vi "AK Befehl Auswerten_v1.1.vi"(10 "Array":string[](array[string])) -> (2 "String für schreiben":string)   [LabVIEW 2020, in "AK-Schnittstelle.lvlib"]
uses:
  AK-Schnittstelle.lvlib
  Aktionen Stoernummern pruefen.ctl
  Aktionen Zustandsfehlerinformation.ctl
  Funktionstasten/Zustaende.ctl
  Funktionstasten/Funktionstasten.lvlib
  Funktionstasten/Betriebsart.ctl
  Funktionstasten/Funktionstasten-Aktion.ctl
  Aktionen Gespeicherte Werte.ctl
  Seiten/Log Konfig/LogKonfig.lvlib
  Seiten/Log Konfig/Aktionen Trigger.ctl
  Seiten/FT-IR/FT-IR.lvlib
  Seiten/FT-IR/FGV FT-IR Gasliste Aktionen.ctl
  Messdaten/Messdaten.lvlib
  Messdaten/Aktionen FGV Messdaten.ctl
  Seiten/System Einstellungen V2/System Einstellungen V2.lvlib
  Seiten/System Einstellungen V2/Aktioen FGV System Konstanten.ctl
  Seiten/Erweiterte Konfig/FGV PID Aktionen.ctl
  Seiten/Erweiterte Konfig/Erweiterte Konfig.lvlib
  Seiten/Erweiterte Konfig/Dichtheitstest.vi
  Allgemein/allgemeine Sub-VIs.lvlib
  cRIO/PC/Kommunikation mit cRIO.lvlib
  Seiten/FT-IR/FGV FT-IR Diagnose Aktionen.ctl
  Seiten/Erweiterte Konfig/Status Dichtheitstest Aktionen.ctl
  Seiten/System Einstellungen V2/Aktioen FGV System.ctl
  AK Namen Aktionen.ctl
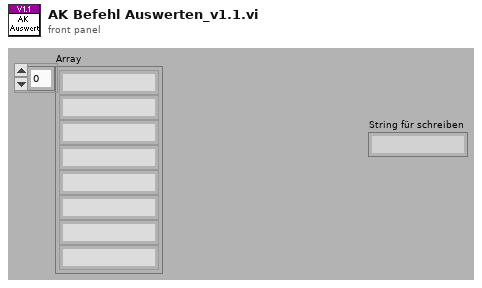
[diagram p1: front panel]
types:
  T1 = typedef "AK-Schnittstelle.lvlib/Aktionen Stoernummern pruefen.ctl" = enum16{"lesen", "prüfen"}
  T2 = typedef "AK-Schnittstelle.lvlib/Aktionen Zustandsfehlerinformation.ctl" = enum16{"OK", "Offline", "Busy", "Syntax Error", "Datenfehler"}
  T3 = typedef "AK-Schnittstelle.lvlib/AK Namen Aktionen.ctl" = enum16{"lesen", "laden", "speichern Namen", "AK Namen", "Liste erstellen", "EKFG erstellen", "speichern EKFG", "EKFG schreiben", "Neuen Eintrag erzeugen"}
  T4 = typedef "AK-Schnittstelle.lvlib/Aktionen Gespeicherte Werte.ctl" = enum16{"lesen", "laden", "speichern", "Seriell", "TCP", "Diverse", "AKTIV", "AK-Namen"}
  T5 = typedef "System Einstellungen V2.lvlib/Aktioen FGV System Konstanten.ctl" = enum16{"lesen", "laden", "speichern", "Sprache"}
  T6 = typedef "System Einstellungen V2.lvlib/Aktioen FGV System.ctl" = enum16{"lesen", "laden", "speichern", "Optionen schreiben", "Zeitstempel", "Reset BMP", "Reset SQP", "Wartung", "Werkseinstellung"}
  T7 = typedef "Messdaten.lvlib/Aktionen FGV Messdaten.ctl" = enum16{"lesen", "schreiben", "löschen", "Mittelwerte", "Komponente"}
  T8 = typedef "Funktionstasten.lvlib/Funktionstasten-Aktion.ctl" = enum16{"Initialisieren", "Zustand setzen", "Taste gedrückt", "Fehler speichern", "Lesen", "Manuell", "Remote", "Bitparallel", "Samplepoint", "Zeit Prüfen", "reset Umschalten"}
  T9 = typedef "FT-IR.lvlib/FGV FT-IR Gasliste Aktionen.ctl" = enum16{"lesen", "Gasliste FT-IR", "Gasliste ausgelesen", "laden", "speichern", "löschen"}
  T10 = typedef "FT-IR.lvlib/FGV FT-IR Diagnose Aktionen.ctl" = enum16{"Lesen", "Diagnose Schreiben", "Min Schreiben", "Max Schreiben"}
  T11 = typedef "Erweiterte Konfig.lvlib/Status Dichtheitstest Aktionen.ctl" = enum16{"lesen", "Zeitstempel", "Daten", "läuft", "Protokolldaten"}
  T12 = typedef "Funktionstasten.lvlib/Zustaende.ctl" = enum16{"Standby", "Pause", "Eco", "Messen", "Kalibrieren", "Spülen Filter", "Spülen Leitung", "Umgebungsluft", "0-Gas", "Cal-Gas", "CG zu PNS", "-------------", "Init 1", "Init 2", "Init 3", "Init 4", "Messen vorbereiten", "Messen durchführen", "Exit"}
  T13 = typedef "Funktionstasten.lvlib/Betriebsart.ctl" = enum16{"Manuell", "Remote", "Bitparallel"}
  T14 = typedef "Funktionstasten.lvlib/Zustaende.ctl" = enum16{"Standby", "Pause", "Eco", "Messen", "Kalibrieren", "Spülen Filter", "Spülen Leitung", "Umgebungsluft", "0-Gas", "Cal-Gas 1", "-------------", "Init 1", "Init 2", "Init 3", "Init 4", "Messen vorbereiten", "Messen durchführen", "Exit"}
  T15 = typedef "LogKonfig.lvlib/Aktionen Trigger.ctl" = enum16{"lesen", "ALLE schreiben", "Trigger prüfen", "Trigger rücksetzen"}
  T16 = typedef "Erweiterte Konfig.lvlib/FGV PID Aktionen.ctl" = enum16{"Lesen", "Schreiben PID", "Schreiben Sonstige", "Dichtheitstest", "Aktionen Dicht.", "Parameter Sensor"}
  T17 = typedef "AK-Schnittstelle.lvlib/Diverse gespeicherte Werte.ctl" = cluster{"Kalibriergaseingang":i16, "SamplePoint":i16, "CalGas zu PNS":i16, "Gas-Reihenfolge":i16[], "Zeit 0-Gas":sgl, "Zeit CalGas":sgl, "AK Befehlssatz":T18}
  T18 = typedef "AK-Schnittstelle.lvlib/AK Befehlssatz.ctl" = enum16{"MEXA", "IAG v1.4", "AVL (Puma)", "PEUS"}
  T19 = typedef "System Einstellungen.lvlib/Optionen.ctl" = cluster{"Störmeldep.":bool, "Betriebszustände":bool, "LN2 Befüllung":bool, "Klimaanlage ?":bool, "AK in ppm":bool, "log Cal-Gas":bool, "log 0-Gas":bool, "log CG zu PNS":bool, "Reserve":bool, "Reserve1":bool, "PNS?":bool, "Container":bool, "Mit N2 spülen":bool, "Span Gas Auswahl":T20}
  T20 = typedef "Funktionstasten.lvlib/Spaneingang.ctl" = u16
  T21 = typedef "String - Ausgabefeld.ctl" = string
  T22 = cluster{"AI0: Durchfluss FT-IR":sgl, "AI1: Druck Ausgang":sgl, "AI2: Umgebungsdruck":sgl, "AI3: Druck FT-IR":sgl, "AI4: Druck CalGas":sgl, "AI5: Reserve":sgl, "AI6: Reserve":sgl, "AI7: Reserve":sgl, "Rohwert Durchfluss FT-IR":sgl, "Rohwert Druck Ausgang":sgl, "Rohwert Umgebungsdruck":sgl, "Rohwert Druck FT-IR":sgl, "Rohwert Durchfluss M":sgl, "TC0: Schaltschrank":sgl, "TC1: Filter":sgl, "TC2: Pumpe":sgl, "TC3: HL BMP zu Filter":sgl, "TC4: HL zu FT-IR":sgl, "TC5: HL Extern SP1":sgl, "TC6: HL Extern SP2":sgl, "TC7: Heizung Extern 1":sgl, "TC8: Heizung Extern 2":sgl, "TC9: Reserve":sgl, "TC10: Reserve":sgl, "TC11: Reserve":sgl, "TC12: FT-IR":sgl, "TC13: Reserve":sgl, "TC14: Reserve":sgl, "TC15: Reserve":sgl}
  T23 = typedef "LogKonfig.lvlib/Element Triggerereignisse.ctl" = cluster{"Trigger verwenden":T24, "Messwert":u16, "kl./gr.":u16, "Wert":sgl, "Puffergröße":sgl}
  T24 = typedef "LogKonfig.lvlib/Auswahlfeld aktiviert-deaktiviert.ctl" = u16
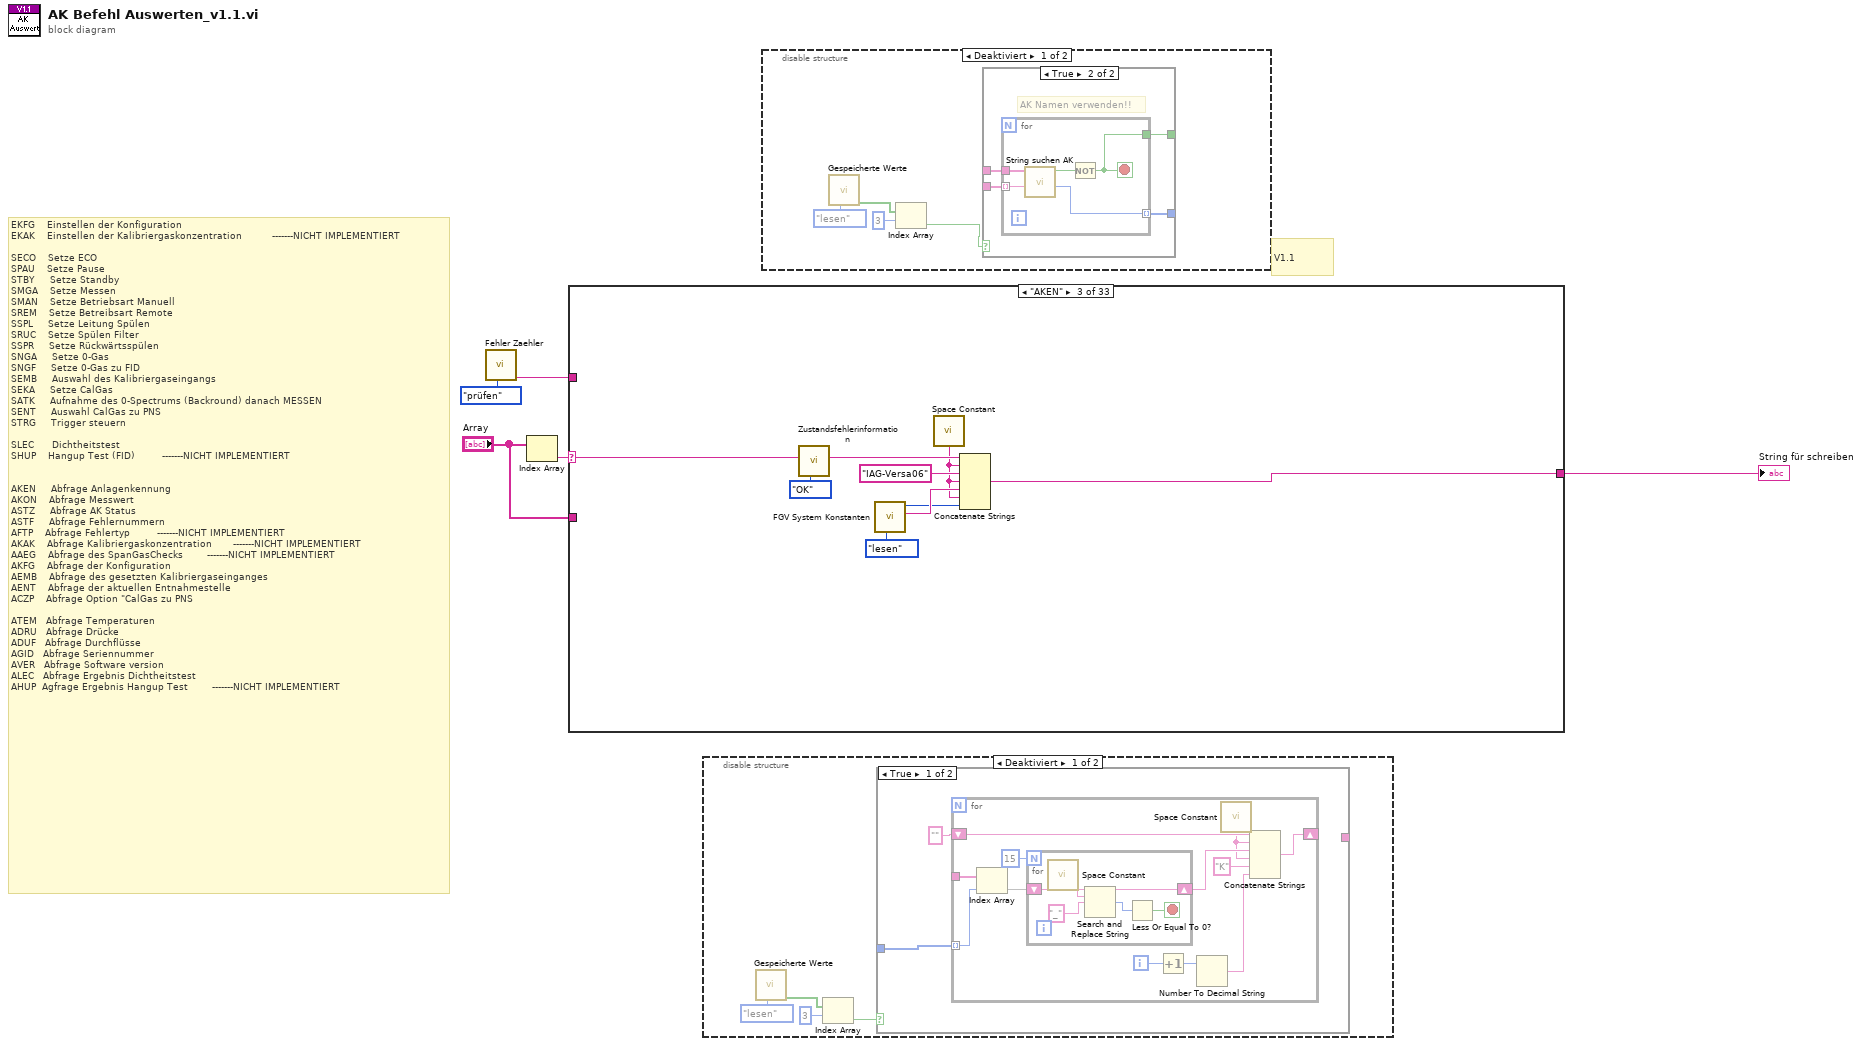
[diagram p0: block diagram]
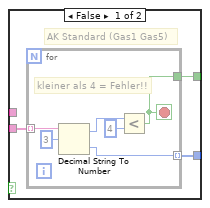
[diagram p2: hidden frame]
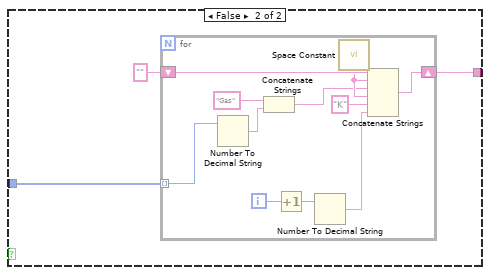
[diagram p4: hidden frame]
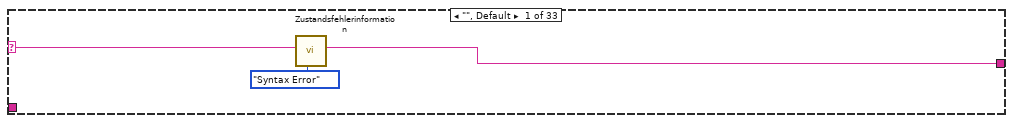
[diagram p6: hidden frame]
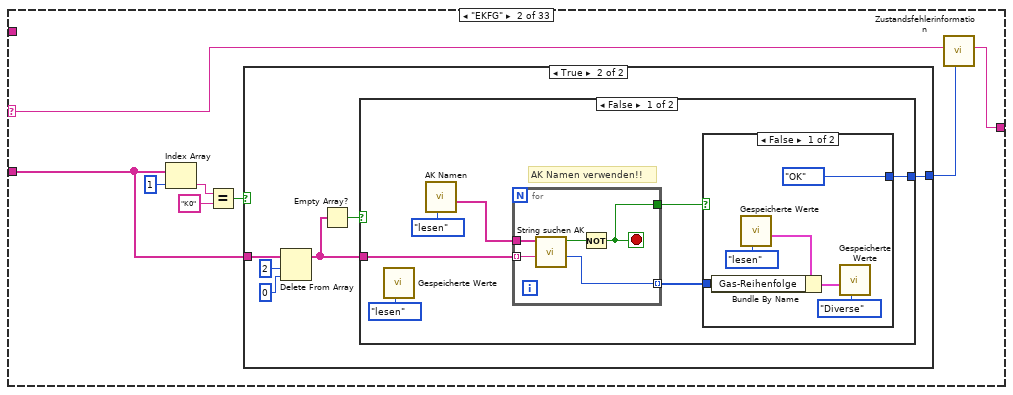
[diagram p7: hidden frame]
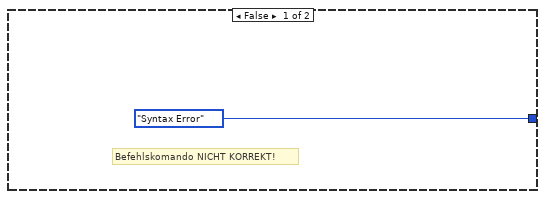
[diagram p8: hidden frame]
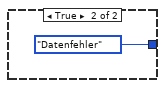
[diagram p9: hidden frame]
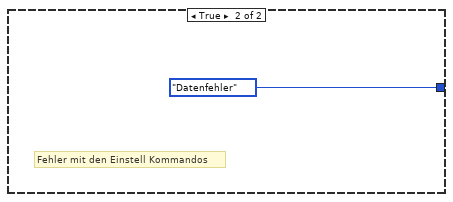
[diagram p10: hidden frame]
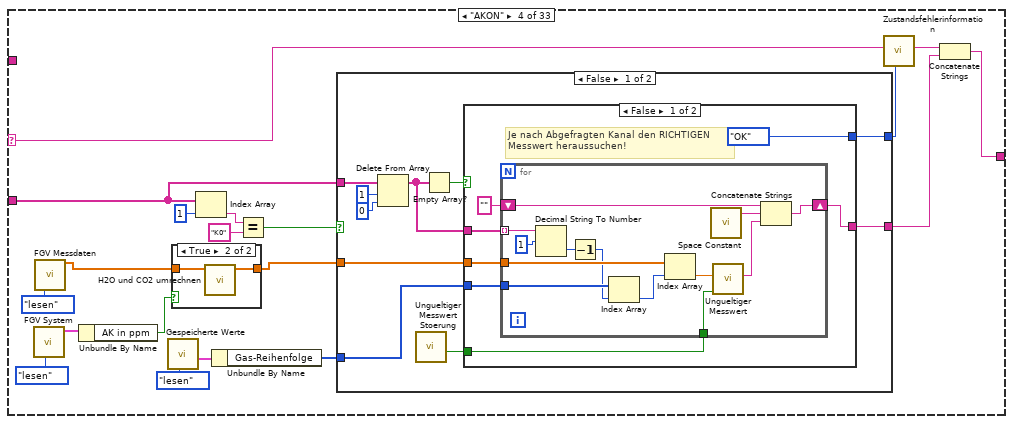
[diagram p11: hidden frame]
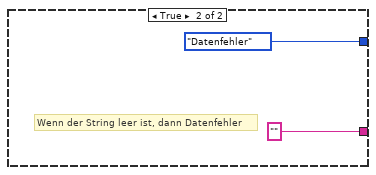
[diagram p13: hidden frame]
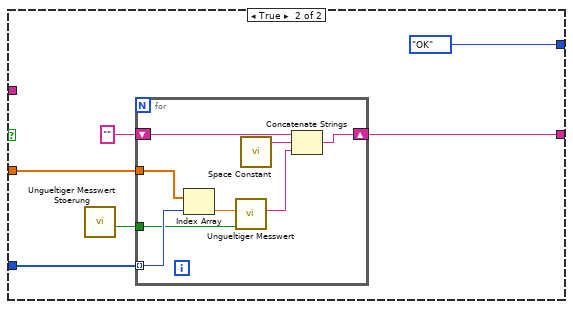
[diagram p14: hidden frame]
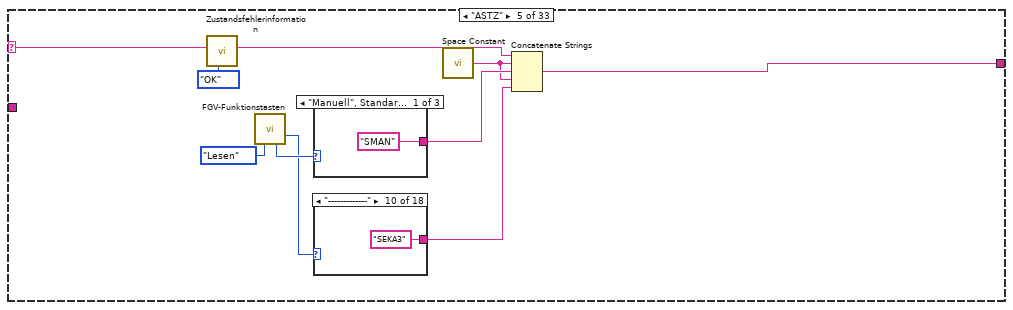
[diagram p15: hidden frame]
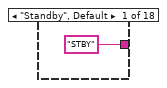
[diagram p16: hidden frame]
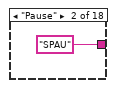
[diagram p17: hidden frame]
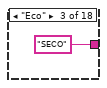
[diagram p18: hidden frame]
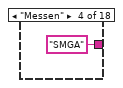
[diagram p19: hidden frame]
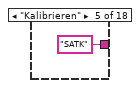
[diagram p20: hidden frame]
diagram:
  # "V1.1"
  # "EKFG    Einstellen der Konfiguration\nEKAK    Einstellen der Kalibriergaskonzentration          -------NICHT IMPLEMENTIERT\n\nSECO    Setze ECO\nSPAU    Setze Pause\nSTBY     Setze Standby\nSMGA    Setze Messen\nSMAN    Setze Betriebsart Manuell\nSREM    Setze Betreibsart Remote\nSSPL     Setze Leitung Spülen\nSRUC    Setze Spülen Filter\nSSPR     Setze Rückwärtsspülen\nSNGA     Setze 0-Gas\nSNGF     Setze 0-Gas zu FID\nSEMB     Auswahl des Kalibriergaseingangs\nSEKA     Setze CalGas\nSATK     Aufnahme des 0-Spectrums (Backround) danach MESSEN\nSENT     Auswahl CalGas zu PNS\nSTRG     Trigger steuern\n\nSLEC      Dichtheitstest\nSHUP    Hangup Test (FID)         -------NICHT IMPLEMENTIERT\n\n\nAKEN     Abfrage Anlagenkennung\nAKON    Abfrage Messwert\nASTZ     Abfrage AK Status\nASTF     Abfrage Fehlernummern\nAFTP    Abfrage Fehlertyp         -------NICHT IMPLEMENTIERT\nAKAK    Abfrage Kalibriergaskonzentration       -------NICHT IMPLEMENTIERT\nAAEG    Abfrage des SpanGasChecks        -------NICHT IMPLEMENTIERT\nAKFG    Abfrage der Konfiguration\nAEMB    Abfrage des gesetzten Kalibriergaseinganges\nAENT    Abfrage der aktuellen Entnahmestelle\nACZP    Abfrage Option \"CalGas zu PNS\n\nATEM   Abfrage Temperaturen\nADRU   Abfrage Drücke\nADUF   Abfrage Durchflüsse\nAGID   Abfrage Seriennummer\nAVER   Abfrage Software version\nALEC   Abfrage Ergebnis Dichtheitstest\nAHUP  Agfrage Ergebnis Hangup Test        -------NICHT IMPLEMENTIERT"
  n1 = call "Fehler Zaehler.vi"("Aktionen"=Aktionen_Stoernummern_pruefen."prüfen") -> ("Fehlerzähler"=w3:string)  [unwired: 7 in, 3 out]
  n2 = Index Array(array="Array") -> (element=w2:string)  [unwired: 1 in]
  n3 = case shown="\"AKEN\"" w2 {
    selector: w2 -> [w7 w15 w49 w70 w128 w148 w159 w189 w198 w207 w223 w246 w260 w267 w274 w289 w298 w301 w304 w307 w317 w327 w331 w341 w345 w347 w360 w365 w386 w405 w409 w431 w470]
    tunnel: [w6 w14 w51 w71 w130 w150 w161 w191 w200 w209 w211 w241 w257 w262 w270 w282 w297 w300 w303 w306 w316 w326 w330 w340 w344 w346 w359 w364 w385 w404 w408 w430 w469] -> w5
    tunnel: w3 -> [_ _ _ _ _ _ _ _ _ _ _ _ _ _ _ _ _ _ _ _ _ _ _ _ _ _ _ _ _ _ _ _ _]
    tunnel: "Array" -> [_ w16 _ w61 _ _ _ _ _ _ _ _ _ _ _ _ _ _ _ _ w309 w319 _ w339 _ _ _ w363 _ _ w407 w429 _]
    frame "", Default {
      n4 = call "Zustandsfehlerinformation.vi"("Aktionen"=Aktionen_Zustandsfehlerinformation."Syntax Error", "String"=w7) -> ("String"=w6:string)  [unwired: 9 in]
    }
    frame "EKFG" {
      n5 = Index Array(array=w16, index=1 ("Index")) -> (element=w12:string)
      n6 = Equal?(x=w12, y="K0") -> (x = y?=w10:bool)
      n7 = case shown="True" w10 {
        tunnel: w16 -> [_ w21]
        tunnel: [Aktionen_Zustandsfehlerinformation."Syntax Error" ("Aktionen") w18] -> w9
        frame False {
          # "Befehlskomando NICHT KORREKT!"
        }
        frame True {
          n8 = Delete From Array(array=w21, length=2 ("Länge"), index=0 ("Index")) -> (array with subset deleted=w20:string[])  [unwired: 1 out]
          n9 = Empty Array?(array=w20) -> (empty?=w19:bool)
          n10 = case shown="False" w19 {
            tunnel: w20 -> [w30 _]
            tunnel: [w27 Aktionen_Zustandsfehlerinformation."Datenfehler" ("Aktionen")] -> w18
            frame False {
              # "AK Namen verwenden!!"
              n11 = call "Gespeicherte Werte.vi"("Aktionen"=Aktionen_Gespeicherte_Werte."lesen") -> ()  [unwired: 6 in, 5 out]
              n12 = call "AK Namen.vi"("Aktionen"=AK_Namen_Aktionen."lesen") -> ("AK Namen"=w24:string[])  [unwired: 7 in, 3 out]
              n13 = for {
                tunnel: w30 -> [w33] mode=indexing
                tunnel: [w32] -> w29 mode=indexing
                tunnel: w24 -> [w34]
                tunnel: [w35] -> w26
                stop <- w35 stop-if-true
                n14 = call "String suchen AK.vi"("gesucht"=w33, "Namen"=w34) -> ("Index"=w32:i32, "Gefunden?"=w31:bool)  [unwired: 8 in]
                n15 = Not(x=w31) -> (.not. x?=w35:bool)
              }
              n16 = case shown="False" w26 {
                tunnel: w29 -> [w40 _]
                tunnel: [Aktionen_Zustandsfehlerinformation."OK" ("Aktionen") Aktionen_Zustandsfehlerinformation."Datenfehler" ("Aktionen")] -> w27
                frame False {
                  n17 = call "Gespeicherte Werte.vi"("Aktionen"=Aktionen_Gespeicherte_Werte."lesen") -> ("Diverse Werte"=w38:T17)  [unwired: 6 in, 4 out]
                  n18 = Bundle By Name(cluster=w38, "Gas-Reihenfolge"=w40) -> (w37:T17)
                  n19 = call "Gespeicherte Werte.vi"("Aktionen"=Aktionen_Gespeicherte_Werte."Diverse", "Diverse Werte"=w37) -> ()  [unwired: 5 in, 5 out]
                }
                frame True {
                }
              }
            }
            frame True {
              # "Fehler mit den Einstell Kommandos"
            }
          }
        }
      }
      n20 = call "Zustandsfehlerinformation.vi"("Aktionen"=w9, "String"=w15) -> ("String"=w14:string)  [unwired: 9 in]
    }
    frame "AKEN" {
      n21 = call "Zustandsfehlerinformation.vi"("Aktionen"=Aktionen_Zustandsfehlerinformation."OK", "String"=w49) -> ("String"=w48:string)  [unwired: 9 in]
      n22 = call "FGV System Konstanten.vi"("Aktionen"=Aktioen_FGV_System_Konstanten."lesen") -> ("LanguageList"=w46:string, "Sprachindex"=w44:u16)  [unwired: 6 in, 3 out]
      n23 = call <vilib>:"Space Constant.vi"() -> ("String"=w45:string)
      n24 = Concatenate Strings(w48, w45, "IAG-Versa06" ("String"), w45, w46, w45, w44) -> (w51:string)
    }
    frame "AKON" {
      n25 = call "FGV System.vi"("Aktionen"=Aktioen_FGV_System."lesen") -> ("Optionen"=w55:T19)  [unwired: 8 in, 2 out]
      n26 = call "FGV Messdaten.vi"("Aktionen"=Aktionen_FGV_Messdaten."lesen") -> ("Aktuelle Messwerte"=w57:sgl[])  [unwired: 6 in, 8 out]
      n27 = Unbundle By Name(w55) -> ("AK in ppm"=w53:bool)
      n28 = call "Gespeicherte Werte.vi"("Aktionen"=Aktionen_Gespeicherte_Werte."lesen") -> ("Diverse Werte"=w59:T17)  [unwired: 6 in, 4 out]
      n29 = case shown="True" w53 {
        tunnel: w57 -> [w72 w74]
        tunnel: [w72 w73] -> w56
        frame False {
        }
        frame True {
          n30 = call "H2O und CO2 umrechnen.vi"("Aktuelle Messwerte"=w74) -> ("Aktuelle Messwerte"=w73:sgl[])  [unwired: 10 in]
        }
      }
      n31 = Index Array(array=w61, index=1 ("Index")) -> (element=w64:string)
      n32 = Unbundle By Name(w59) -> ("Gas-Reihenfolge"=w67:i16[])
      n33 = Equal?(x=w64, y="K0") -> (x = y?=w62:bool)
      n34 = case shown="False" w62 {
        tunnel: w67 -> [w78 w112]
        tunnel: [w76 w110] -> w66
        tunnel: w56 -> [w77 w109]
        tunnel: w61 -> [w82 _]
        tunnel: [w80 Aktionen_Zustandsfehlerinformation."OK" ("Aktionen")] -> w60
        frame False {
          n35 = Delete From Array(array=w82, length=1 ("Länge"), index=0 ("Index")) -> (array with subset deleted=w79:string[])  [unwired: 1 out]
          n36 = call "Ungueltiger Messwert Stoerung.vi"() -> ("Störung Messgerät"=w75:bool)  [unwired: 11 in]
          n37 = Empty Array?(array=w79) -> (empty?=w81:bool)
          n38 = case shown="False" w81 {
            tunnel: [Aktionen_Zustandsfehlerinformation."OK" ("Aktionen") Aktionen_Zustandsfehlerinformation."Datenfehler" ("Aktionen")] -> w80
            tunnel: w79 -> [w90 _]
            tunnel: w78 -> [w89 _]
            tunnel: w77 -> [w88 _]
            tunnel: [w87 ""] -> w76
            tunnel: w75 -> [w85 _]
            frame False {
              # "Je nach Abgefragten Kanal den RICHTIGEN\nMesswert heraussuchen!"
              n39 = for {
                tunnel: w90 -> [w104] mode=indexing
                tunnel: w89 -> [w102]
                tunnel: w88 -> [w101]
                shift-right: [w100] -> w87
                shift-left: "" -> [w99]
                tunnel: w85 -> [w93]
                n40 = Decimal String To Number(string=w104, offset=1 ("Offset (0)")) -> (number=w98:i32)  [unwired: 1 in, 1 out]
                n41 = Decrement(x=w98) -> (x-1=w97:i32)
                n42 = Index Array(array=w102, index=w97) -> (element=w95:i16)
                n43 = Index Array(array=w101, index=w95) -> (element=w94:sgl)
                n44 = call <vilib>:"Space Constant.vi"() -> ("String"=w96:string)
                n45 = call "Ungueltiger Messwert.vi"("Stöung Messgerät"=w93, "Messwert"=w94) -> ("Messwert String"=w92:string)  [unwired: 9 in]
                n46 = Concatenate Strings(w99, w96, w92) -> (w100:string)
              }
            }
            frame True {
              # "Wenn der String leer ist, dann Datenfehler"
            }
          }
        }
        frame True {
          n47 = call "Ungueltiger Messwert Stoerung.vi"() -> ("Störung Messgerät"=w107:bool)  [unwired: 11 in]
          n48 = for {
            tunnel: w112 -> [w116] mode=indexing
            shift-right: [w120] -> w110
            shift-left: "" -> [w119]
            tunnel: w109 -> [w118]
            tunnel: w107 -> [w114]
            n49 = Index Array(array=w118, index=w116) -> (element=w115:sgl)
            n50 = call "Ungueltiger Messwert.vi"("Stöung Messgerät"=w114, "Messwert"=w115) -> ("Messwert String"=w113:string)  [unwired: 9 in]
            n51 = call <vilib>:"Space Constant.vi"() -> ("String"=w117:string)
            n52 = Concatenate Strings(w119, w117, w113) -> (w120:string)
          }
        }
      }
      n53 = call "Zustandsfehlerinformation.vi"("Aktionen"=w60, "String"=w70) -> ("String"=w69:string)  [unwired: 9 in]
      n54 = Concatenate Strings(w69, w66) -> (w71:string)
    }
    frame "ASTZ" {
      n55 = call "Zustandsfehlerinformation.vi"("Aktionen"=Aktionen_Zustandsfehlerinformation."OK", "String"=w128) -> ("String"=w127:string)  [unwired: 9 in]
      n56 = call "FGV-Funktionstasten.vi"("Aktion"=Funktionstasten-Aktion."Lesen") -> ("ausgewählte Funktion"=w123:T12, "Betriebsart"=w125:T13)  [unwired: 7 in, 6 out]
      n57 = case shown="\"Manuell\", Standard" w125 {
        tunnel: ["SMAN" ("String") "SREM" ("String") "SBIT" ("String")] -> w124
        frame "Manuell", Default {
        }
        frame "Remote" {
        }
        frame "Bitparallel" {
        }
      }
      n58 = case shown="\"-------------\"" w123 {
        tunnel: ["STBY" ("String") "SPAU" ("String") "SECO" ("String") "SMGA" ("String") "SATK" ("String") "SRUC" ("String") "SSPL" ("String") "SNGA" ("String") "SEKA1" ("String") "SEKA3" ("String") _ _ _ _ _ _ _ _] -> w121
        frame "Standby", Default {
        }
        frame "Pause" {
        }
        frame "Eco" {
        }
        frame "Messen" {
        }
        frame "Kalibrieren" {
        }
        frame "Spülen Filter" {
        }
        frame "Spülen Leitung" {
        }
        frame "0-Gas" {
        }
        frame "Cal-Gas" {
        }
        frame "-------------" {
        }
        frame "-------------" {
        }
        frame "Init 1" {
        }
        frame "Init 2" {
        }
        frame "Init 3" {
        }
        frame "Init 4" {
        }
        frame "Messen vorbereiten" {
        }
        frame "Messen durchführen" {
        }
        frame "Exit" {
        }
      }
      n59 = call <vilib>:"Space Constant.vi"() -> ("String"=w122:string)
      n60 = Concatenate Strings(w127, w122, w124, w122, w121) -> (w130:string)
    }
    frame "ASTF" {
      n61 = call "Zustandsfehlerinformation.vi"("Aktionen"=Aktionen_Zustandsfehlerinformation."OK", "String"=w148) -> ("String"=w147:string)  [unwired: 9 in]
      n62 = call "Fehler Zaehler.vi"("Aktionen"=Aktionen_Stoernummern_pruefen."lesen") -> ("Fehler Nummern"=w145:string)  [unwired: 7 in, 3 out]
      n63 = call <vilib>:"Space Constant.vi"() -> ("String"=w144:string)
      n64 = Concatenate Strings(w147, w144, w145) -> (w150:string)
    }
    frame "AKFG" {
      n65 = call "Gespeicherte Werte.vi"("Aktionen"=Aktionen_Gespeicherte_Werte."lesen") -> ("Diverse Werte"=w156:T17)  [unwired: 6 in, 4 out]
      n66 = Unbundle By Name(w156) -> ("Gas-Reihenfolge"=w154:i16[])
      n67 = disable-structure shown="Deaktiviert" {
        disable-tunnel: [w180 _] -> _
        frame Disabled {
          n68 = call "FGV Gasliste.vi"("Aktionen"=FGV_FT-IR_Gasliste_Aktionen."lesen") -> ("Aktuelle Gasliste gesamt"=w180:T21[])  [unwired: 8 in, 2 out]
        }
        frame Enabled {
        }
      }
      n69 = call "AK Namen.vi"("Aktionen"=AK_Namen_Aktionen."lesen") -> ("AK Namen"=w151:string[])  [unwired: 7 in, 3 out]
      n70 = for {
        tunnel: w154 -> [w170] mode=indexing
        shift-right: [w173] -> w153
        shift-left: "" -> [w172]
        tunnel: w151 -> [w171]
        i -> [w163]
        n71 = Index Array(array=w171, index=w170) -> (element=w168:string)
        n72 = for {
          N: 15 -> [_]
          shift-right: [w178] -> w167
          shift-left: w168 -> [w179]
          stop <- w176 stop-if-true
          n73 = call <vilib>:"Space Constant.vi"() -> ("String"=w175:string)
          n74 = Search and Replace String(input string=w179, search string=w175, replace string="_") -> (result string=w178:string, number of replacements=w177:i32)  [unwired: 5 in, 2 out]
          n75 = Less Or Equal To 0?(x=w177) -> (x <= 0?=w176:bool)
        }
        n76 = Increment(x=w163) -> (x+1=w165:i32)
        n77 = Number To Decimal String(number=w165) -> (decimal integer string=w162:string)  [unwired: 1 in]
        n78 = call <vilib>:"Space Constant.vi"() -> ("String"=w166:string)
        n79 = Concatenate Strings(w172, w166, w167, w166, "K" ("String"), w162) -> (w173:string)
      }
      n80 = call "Zustandsfehlerinformation.vi"("Aktionen"=Aktionen_Zustandsfehlerinformation."OK", "String"=w159) -> ("String"=w158:string)  [unwired: 9 in]
      n81 = Concatenate Strings(w158, w153) -> (w161:string)
    }
    frame "AEMB" {
      n82 = call "Zustandsfehlerinformation.vi"("Aktionen"=Aktionen_Zustandsfehlerinformation."OK", "String"=w189) -> ("String"=w188:string)  [unwired: 9 in]
      n83 = call "Gespeicherte Werte.vi"("Aktionen"=Aktionen_Gespeicherte_Werte."lesen") -> ("Diverse Werte"=w182:T17)  [unwired: 6 in, 4 out]
      n84 = Unbundle By Name(w182) -> ("Kalibriergaseingang"=w186:i16)
      n85 = call <vilib>:"Space Constant.vi"() -> ("String"=w183:string)
      n86 = Number To Decimal String(number=w186) -> (decimal integer string=w184:string)  [unwired: 1 in]
      n87 = Concatenate Strings(w188, w183, "M" ("String"), w184) -> (w191:string)
    }
    frame "AENT" {
      n88 = call "Zustandsfehlerinformation.vi"("Aktionen"=Aktionen_Zustandsfehlerinformation."OK", "String"=w198) -> ("String"=w197:string)  [unwired: 9 in]
      n89 = call "FGV-Funktionstasten.vi"("Aktion"=Funktionstasten-Aktion."Lesen") -> ("Samplepoint"=w192:u16)  [unwired: 7 in, 7 out]
      n90 = call <vilib>:"Space Constant.vi"() -> ("String"=w194:string)
      n91 = Number To Decimal String(number=w192) -> (decimal integer string=w195:string)  [unwired: 1 in]
      n92 = Concatenate Strings(w197, w194, "M" ("String"), w195) -> (w200:string)
    }
    frame "ACZP" {
      n93 = call "Zustandsfehlerinformation.vi"("Aktionen"=Aktionen_Zustandsfehlerinformation."OK", "String"=w207) -> ("String"=w206:string)  [unwired: 9 in]
      n94 = call "Gespeicherte Werte.vi"("Aktionen"=Aktionen_Gespeicherte_Werte."lesen") -> ("Diverse Werte"=w201:T17)  [unwired: 6 in, 4 out]
      n95 = Unbundle By Name(w201) -> ("CalGas zu PNS"=w204:i16)
      n96 = call <vilib>:"Space Constant.vi"() -> ("String"=w202:string)
      n97 = Number To Decimal String(number=w204) -> (decimal integer string=w203:string)  [unwired: 1 in]
      n98 = Concatenate Strings(w206, w202, w203) -> (w209:string)
    }
    frame "ATEM" {
      n99 = call "Zustandsfehlerinformation.vi"("Aktionen"=Aktionen_Zustandsfehlerinformation."OK", "String"=w223) -> ("String"=w210:string)  [unwired: 9 in]
      n100 = call "FGV cRIO-Daten.vi"("Aktion"=enum16{"lesen", "schreiben"}."lesen") -> ("Analog Input"=w221:T22)  [unwired: 6 in, 8 out]
      n101 = Unbundle By Name(w221) -> ("TC1: Filter"=w218:sgl, "TC2: Pumpe"=w217:sgl, "TC3: HL BMP zu Filter"=w216:sgl, "TC4: HL zu FT-IR"=w215:sgl, "TC5: HL Extern SP1"=w214:sgl, "TC0: Schaltschrank"=w213:sgl)
      n102 = call "FGV FT-IR Diagnosewerte.vi"("Aktionen"=FGV_FT-IR_Diagnose_Aktionen."Lesen") -> ("Temperatur"=w219:dbl)  [unwired: 5 in, 5 out]
      n103 = Build Array(w219, w218, w217, w216, w215, w214, w213) -> (w212:dbl[])
      n104 = for {
        tunnel: w212 -> [w230] mode=indexing
        shift-right: [w225] -> w211
        shift-left: w210 -> [w228]
        n105 = Number To Fractional String(number=w230, precision (6)=i16 1 ("Genauigkeit (6)")) -> (F-format string=w226:string)  [unwired: 2 in]
        n106 = call <vilib>:"Space Constant.vi"() -> ("String"=w227:string)
        n107 = Concatenate Strings(w228, w227, w226) -> (w225:string)
      }
    }
    frame "ADRU" {
      n108 = call "Zustandsfehlerinformation.vi"("Aktionen"=Aktionen_Zustandsfehlerinformation."OK", "String"=w246) -> ("String"=w240:string)  [unwired: 9 in]
      n109 = call "FGV cRIO-Daten.vi"("Aktion"=enum16{"lesen", "schreiben"}."lesen") -> ("Analog Input"=w244:T22)  [unwired: 6 in, 8 out]
      n110 = Unbundle By Name(w244) -> ("AI1: Druck Ausgang"=w236:sgl, "AI4: Druck CalGas"=w234:sgl)
      n111 = call "FGV FT-IR Diagnosewerte.vi"("Aktionen"=FGV_FT-IR_Diagnose_Aktionen."Lesen") -> ("Druck"=w238:dbl)  [unwired: 5 in, 5 out]
      n112 = Number To Fractional String(number=w238, precision (6)=i16 3 ("Genauigkeit (6)")) -> (F-format string=w233:string)  [unwired: 2 in]
      n113 = Number To Fractional String(number=w236, precision (6)=i16 0 ("Genauigkeit (6)")) -> (F-format string=w231:string)  [unwired: 2 in]
      n114 = Number To Fractional String(number=w234, precision (6)=i16 1 ("Genauigkeit (6)")) -> (F-format string=w232:string)  [unwired: 2 in]
      n115 = Build Array(w233, w231, w232) -> (w242:string[])
      n116 = for {
        tunnel: w242 -> [w248] mode=indexing
        shift-right: [w249] -> w241
        shift-left: w240 -> [w251]
        n117 = call <vilib>:"Space Constant.vi"() -> ("String"=w250:string)
        n118 = Concatenate Strings(w251, w250, w248) -> (w249:string)
      }
    }
    frame "ADUF" {
      n119 = call "Zustandsfehlerinformation.vi"("Aktionen"=Aktionen_Zustandsfehlerinformation."OK", "String"=w260) -> ("String"=w256:string)  [unwired: 9 in]
      n120 = call "FGV cRIO-Daten.vi"("Aktion"=enum16{"lesen", "schreiben"}."lesen") -> ("Analog Input"=w259:T22)  [unwired: 6 in, 8 out]
      n121 = Unbundle By Name(w259) -> ("AI0: Durchfluss FT-IR"=w255:sgl)
      n122 = Number To Fractional String(number=w255, precision (6)=i16 1 ("Genauigkeit (6)")) -> (F-format string=w252:string)  [unwired: 2 in]
      n123 = call <vilib>:"Space Constant.vi"() -> ("String"=w253:string)
      n124 = Concatenate Strings(w256, w253, w252) -> (w257:string)
    }
    frame "AGID" {
      n125 = call "Zustandsfehlerinformation.vi"("Aktionen"=Aktionen_Zustandsfehlerinformation."OK", "String"=w267) -> ("String"=w264:string)  [unwired: 9 in]
      n126 = call "FGV System Konstanten.vi"("Aktionen"=Aktioen_FGV_System_Konstanten."lesen") -> ("LanguageList"=w263:string)  [unwired: 6 in, 4 out]
      n127 = call <vilib>:"Space Constant.vi"() -> ("String"=w266:string)
      n128 = Concatenate Strings(w264, w266, w263) -> (w262:string)
    }
    frame "AVER" {
      n129 = call "Zustandsfehlerinformation.vi"("Aktionen"=Aktionen_Zustandsfehlerinformation."OK", "String"=w274) -> ("String"=w271:string)  [unwired: 9 in]
      n130 = call "FGV System Konstanten.vi"("Aktionen"=Aktioen_FGV_System_Konstanten."lesen") -> ("Sprachindex"=w269:u16)  [unwired: 6 in, 4 out]
      n131 = call <vilib>:"Space Constant.vi"() -> ("String"=w273:string)
      n132 = Concatenate Strings(w271, w273, w269) -> (w270:string)
    }
    frame "ALEC" {
      n133 = call "Zustandsfehlerinformation.vi"("Aktionen"=Aktionen_Zustandsfehlerinformation."OK", "String"=w289) -> ("String"=w288:string)  [unwired: 9 in]
      n134 = call "Status Dichtheitstest.vi"("Aktionen"=Status_Dichtheitstest_Aktionen."lesen") -> ("Fehler"=w277:bool, "läuft?"=w281:bool, "Anstieg"=w286:sgl)  [unwired: 6 in, 2 out]
      n135 = Or(x=w281, y=w277) -> (x .or. y?=w280:bool)
      n136 = Number To Decimal String(number=w286) -> (decimal integer string=w285:string)  [unwired: 1 in]
      n137 = call <vilib>:"Space Constant.vi"() -> ("String"=w284:string)
      n138 = Concatenate Strings(w288, w284, w285) -> (w283:string)
      n139 = Select(t="error", s=w277, f="busy") -> (s? t:f=w276:string)
      n140 = case shown="True" w280 {
        tunnel: w283 -> [w291 w294]
        tunnel: [w291 w292] -> w282
        tunnel: w276 -> [_ w293]
        frame False {
        }
        frame True {
          n141 = call <vilib>:"Space Constant.vi"() -> ("String"=w295:string)
          n142 = Concatenate Strings(w294, w295, w293) -> (w292:string)
        }
      }
    }
    frame "SECO" {
      n143 = call "Setze Zustand.vi"("AK Befehl"=w298, "Zustand"=Zustaende."Eco") -> ("Antwort String"=w297:string)  [unwired: 8 in, 1 out]
    }
    frame "SPAU" {
      n144 = call "Setze Zustand.vi"("AK Befehl"=w301, "Zustand"=Zustaende."Pause") -> ("Antwort String"=w300:string)  [unwired: 8 in, 1 out]
    }
    frame "STBY" {
      n145 = call "Setze Zustand.vi"("AK Befehl"=w304, "Zustand"=Zustaende."Standby") -> ("Antwort String"=w303:string)  [unwired: 8 in, 1 out]
    }
    frame "SMGA" {
      n146 = call "Setze Zustand.vi"("AK Befehl"=w307, "Zustand"=Zustaende."Messen") -> ("Antwort String"=w306:string)  [unwired: 8 in, 1 out]
    }
    frame "SSPL" {
      n147 = Index Array(array=w309, index=2 ("Index")) -> (element=w313:string)
      n148 = Decimal String To Number(string=w313) -> (number=w312:i32)  [unwired: 2 in, 1 out]
      n149 = Divide(x=w312, y=10) -> (x/y=w310:dbl)
      n150 = To Single Precision Float(number=w310) -> (single precision float=w308:sgl)
      n151 = call "Setze Zustand.vi"("Zeit"=w308, "AK Befehl"=w317, "Zustand"=Zustaende."Spülen Leitung") -> ("Antwort String"=w316:string)  [unwired: 7 in, 1 out]
    }
    frame "SRUC" {
      n152 = Index Array(array=w319, index=2 ("Index")) -> (element=w323:string)
      n153 = Decimal String To Number(string=w323) -> (number=w322:i32)  [unwired: 2 in, 1 out]
      n154 = Divide(x=w322, y=10) -> (x/y=w320:dbl)
      n155 = To Single Precision Float(number=w320) -> (single precision float=w318:sgl)
      n156 = call "Setze Zustand.vi"("Zeit"=w318, "AK Befehl"=w327, "Zustand"=Zustaende."Spülen Filter") -> ("Antwort String"=w326:string)  [unwired: 7 in, 1 out]
    }
    frame "SSPR" {
      n157 = call "Setze Zustand.vi"("Befehl nicht vorhanden!"=TRUE, "AK Befehl"=w331, "Zustand"=Zustaende."Standby") -> ("Antwort String"=w330:string)  [unwired: 7 in, 1 out]
    }
    frame "SNGA" {
      n158 = Index Array(array=w339, index=2 ("Index")) -> (element=w337:string)
      n159 = Decimal String To Number(string=w337) -> (number=w336:i32)  [unwired: 2 in, 1 out]
      n160 = Divide(x=w336, y=10) -> (x/y=w334:dbl)
      n161 = To Single Precision Float(number=w334) -> (single precision float=w332:sgl)
      n162 = call "Setze Zustand.vi"("Zeit"=w332, "AK Befehl"=w341, "Zustand"=Zustaende."0-Gas") -> ("Antwort String"=w340:string)  [unwired: 7 in, 1 out]
    }
    frame "SNGF" {
      n163 = call "Setze Zustand.vi"("Befehl nicht vorhanden!"=TRUE, "AK Befehl"=w345, "Zustand"=Zustaende."Standby") -> ("Antwort String"=w344:string)  [unwired: 7 in, 1 out]
    }
    frame "SMAN" {
      n164 = call "FGV-Funktionstasten.vi"("Aktion"=Funktionstasten-Aktion."Lesen") -> ("Betriebsart"=w351:T13)  [unwired: 7 in, 7 out]
      n165 = Equal?(x=w351, y=Betriebsart."Remote" ("Betriebsart")) -> (x = y?=w348:bool)
      n166 = case shown="True" w348 {
        tunnel: w347 -> [w354 w357]
        tunnel: [w352 w356] -> w346
        frame False {
          n167 = call "Zustandsfehlerinformation.vi"("Aktionen"=Aktionen_Zustandsfehlerinformation."Offline", "String"=w354) -> ("String"=w352:string)  [unwired: 9 in]
        }
        frame True {
          n168 = call "Zustandsfehlerinformation.vi"("Aktionen"=Aktionen_Zustandsfehlerinformation."OK", "String"=w357) -> ("String"=w356:string)  [unwired: 9 in]
          n169 = call "FGV-Funktionstasten.vi"("Aktion"=Funktionstasten-Aktion."Manuell") -> ()  [unwired: 7 in, 8 out]
        }
      }
    }
    frame "SREM" {
      n170 = call "Zustandsfehlerinformation.vi"("Aktionen"=Aktionen_Zustandsfehlerinformation."OK", "String"=w360) -> ("String"=w359:string)  [unwired: 9 in]
      n171 = call "FGV-Funktionstasten.vi"("Aktion"=Funktionstasten-Aktion."Remote") -> ()  [unwired: 7 in, 8 out]
    }
    frame "SEMB" {
      n172 = call "FGV-Funktionstasten.vi"("Aktion"=Funktionstasten-Aktion."Lesen") -> ("Betriebsart"=w368:T13)  [unwired: 7 in, 7 out]
      n173 = Equal?(x=w368, y=Betriebsart."Remote" ("Betriebsart")) -> (x = y?=w369:bool)
      n174 = case shown="True" w369 {
        tunnel: w365 -> [w371 w383]
        tunnel: [w370 w382] -> w364
        tunnel: w363 -> [_ w381]
        frame False {
          n175 = call "Zustandsfehlerinformation.vi"("Aktionen"=Aktionen_Zustandsfehlerinformation."Offline", "String"=w371) -> ("String"=w370:string)  [unwired: 9 in]
        }
        frame True {
          n176 = Index Array(array=w381, index=2 ("Index")) -> (element=w379:string)
          n177 = call "Zustandsfehlerinformation.vi"("Aktionen"=Aktionen_Zustandsfehlerinformation."OK", "String"=w383) -> ("String"=w382:string)  [unwired: 9 in]
          n178 = Decimal String To Number(string=w379, offset=1 ("Offset (0)")) -> (number=w375:i32)  [unwired: 1 in, 1 out]
          n179 = call "Gespeicherte Werte.vi"("Aktionen"=Aktionen_Gespeicherte_Werte."lesen") -> ("Diverse Werte"=w374:T17)  [unwired: 6 in, 4 out]
          n180 = Bundle By Name(cluster=w374, "Kalibriergaseingang"=w375) -> (w373:T17)
          n181 = call "Gespeicherte Werte.vi"("Aktionen"=Aktionen_Gespeicherte_Werte."Diverse", "Diverse Werte"=w373) -> ()  [unwired: 5 in, 5 out]
        }
      }
    }
    frame "SEKA" {
      n182 = call "FGV-Funktionstasten.vi"("Aktion"=Funktionstasten-Aktion."Lesen") -> ("Betriebsart"=w389:T13)  [unwired: 7 in, 7 out]
      n183 = Equal?(x=w389, y=Betriebsart."Remote" ("Betriebsart")) -> (x = y?=w390:bool)
      n184 = case shown="True" w390 {
        tunnel: w386 -> [w392 w396]
        tunnel: [w391 w395] -> w385
        frame False {
          n185 = call "Zustandsfehlerinformation.vi"("Aktionen"=Aktionen_Zustandsfehlerinformation."Offline", "String"=w392) -> ("String"=w391:string)  [unwired: 9 in]
        }
        frame True {
          n186 = call "Gespeicherte Werte.vi"("Aktionen"=Aktionen_Gespeicherte_Werte."lesen") -> ("Diverse Werte"=w398:T17)  [unwired: 6 in, 4 out]
          n187 = Unbundle By Name(w398) -> ("Kalibriergaseingang"=w397:i16)
          n188 = case shown="3" w397 {
            tunnel: [Zustaende."Standby" ("Zustand") Zustaende."Cal-Gas 1" ("Zustand") Zustaende."-------------" ("Zustand") Zustaende."Init 1" ("Zustand")] -> w394
            frame 0, Default {
            }
            frame 1 {
            }
            frame 2 {
            }
            frame 3 {
            }
          }
          n189 = call "Setze Zustand.vi"("AK Befehl"=w396, "Zustand"=w394) -> ("Antwort String"=w395:string)  [unwired: 8 in, 1 out]
        }
      }
    }
    frame "SATK" {
      n190 = call "Setze Zustand.vi"("AK Befehl"=w405, "Zustand"=Zustaende."Kalibrieren") -> ("Antwort String"=w404:string)  [unwired: 8 in, 1 out]
    }
    frame "SENT" {
      n191 = call "FGV-Funktionstasten.vi"("Aktion"=Funktionstasten-Aktion."Lesen") -> ("Betriebsart"=w412:T13)  [unwired: 7 in, 7 out]
      n192 = Equal?(x=w412, y=Betriebsart."Remote" ("Betriebsart")) -> (x = y?=w413:bool)
      n193 = case shown="True" w413 {
        tunnel: w409 -> [w415 w427]
        tunnel: [w414 w426] -> w408
        tunnel: w407 -> [_ w425]
        frame False {
          n194 = call "Zustandsfehlerinformation.vi"("Aktionen"=Aktionen_Zustandsfehlerinformation."Offline", "String"=w415) -> ("String"=w414:string)  [unwired: 9 in]
        }
        frame True {
          n195 = Index Array(array=w425, index=2 ("Index")) -> (element=w423:string)
          n196 = call "Zustandsfehlerinformation.vi"("Aktionen"=Aktionen_Zustandsfehlerinformation."OK", "String"=w427) -> ("String"=w426:string)  [unwired: 9 in]
          n197 = Decimal String To Number(string=w423) -> (number=w417:i32)  [unwired: 2 in, 1 out]
          n198 = call "FGV-Funktionstasten.vi"("Samplepoint"=w417, "Aktion"=Funktionstasten-Aktion."Samplepoint") -> ()  [unwired: 6 in, 8 out]
          n199 = call "Gespeicherte Werte.vi"("Aktionen"=Aktionen_Gespeicherte_Werte."lesen") -> ("Diverse Werte"=w420:T17)  [unwired: 6 in, 4 out]
          n200 = Bundle By Name(cluster=w420, "SamplePoint"=w417) -> (w419:T17)
          n201 = call "Gespeicherte Werte.vi"("Aktionen"=Aktionen_Gespeicherte_Werte."Diverse", "Diverse Werte"=w419) -> ()  [unwired: 5 in, 5 out]
        }
      }
    }
    frame "STRG" {
      n202 = call "FGV-Funktionstasten.vi"("Aktion"=Funktionstasten-Aktion."Lesen") -> ("Betriebsart"=w434:T13)  [unwired: 7 in, 7 out]
      n203 = Equal?(x=w434, y=Betriebsart."Remote" ("Betriebsart")) -> (x = y?=w435:bool)
      n204 = case shown="False" w435 {
        tunnel: w431 -> [w437 w444]
        tunnel: [w436 w443] -> w430
        tunnel: w429 -> [_ w442]
        frame False {
          n205 = call "Zustandsfehlerinformation.vi"("Aktionen"=Aktionen_Zustandsfehlerinformation."Offline", "String"=w437) -> ("String"=w436:string)  [unwired: 9 in]
        }
        frame True {
          n206 = Index Array(array=w442, index=2 ("Index")) -> (element=w440:string)
          n207 = Empty String/Path?(string/path=w440) -> (empty?=w439:bool)
          n208 = case shown="True" w439 {
            tunnel: w444 -> [w451 w464]
            tunnel: [w450 w463] -> w443
            tunnel: w440 -> [w449 _]
            frame False {
              n209 = Decimal String To Number(string=w449) -> (number=w446:i32)  [unwired: 2 in, 1 out]
              n210 = In Range and Coerce(upper limit=2 ("Obergrenze"), x=w446, lower limit=0 ("Untergrenze")) -> (In Range?=w445:bool)  [unwired: 1 out]
              n211 = case shown="True" w445 {
                tunnel: w451 -> [w453 w461]
                tunnel: [w452 w460] -> w450
                tunnel: w446 -> [_ w455]
                frame False {
                  n212 = call "Zustandsfehlerinformation.vi"("Aktionen"=Aktionen_Zustandsfehlerinformation."Datenfehler", "String"=w453) -> ("String"=w452:string)  [unwired: 9 in]
                }
                frame True {
                  # "Wenn informationen da sind, dann übergeben!"
                  n213 = call "FGV Trigger.vi"("Aktion"=Aktionen_Trigger."lesen") -> ("Triggerereignis neu"=w457:T23)  [unwired: 7 in, 3 out]
                  n214 = Bundle By Name(cluster=w457, "Trigger verwenden"=w455) -> (w456:T23)
                  n215 = call "Zustandsfehlerinformation.vi"("Aktionen"=Aktionen_Zustandsfehlerinformation."OK", "String"=w461) -> ("String"=w460:string)  [unwired: 9 in]
                  n216 = call "FGV Trigger.vi"("Aktion"=Aktionen_Trigger."ALLE schreiben", "Triggerereignis"=w456) -> ()  [unwired: 6 in, 4 out]
                }
              }
            }
            frame True {
              # "Wenn nur STRG dann Trigger setzen!!!"
              n217 = call "FGV Trigger.vi"("Aktion"=Aktionen_Trigger."Trigger prüfen", "Trigger setzen"=TRUE) -> ()  [unwired: 6 in, 4 out]
              n218 = call "Zustandsfehlerinformation.vi"("Aktionen"=Aktionen_Zustandsfehlerinformation."OK", "String"=w464) -> ("String"=w463:string)  [unwired: 9 in]
            }
          }
        }
      }
    }
    frame "SLEC" {
      n219 = call "FGV-Funktionstasten.vi"("Aktion"=Funktionstasten-Aktion."Lesen") -> ("ausgewählte Funktion"=w468:T12, "Betriebsart"=w473:T13)  [unwired: 7 in, 6 out]
      n220 = Equal?(x=w473, y=Betriebsart."Remote" ("Betriebsart")) -> (x = y?=w474:bool)
      n221 = case shown="True" w474 {
        tunnel: w470 -> [w476 w482]
        tunnel: [w475 w481] -> w469
        tunnel: w468 -> [_ w480]
        frame False {
          n222 = call "Zustandsfehlerinformation.vi"("Aktionen"=Aktionen_Zustandsfehlerinformation."Offline", "String"=w476) -> ("String"=w475:string)  [unwired: 9 in]
        }
        frame True {
          n223 = Equal?(x=w480, y=Zustaende."Standby") -> (x = y?=w478:bool)
          n224 = case shown="True" w478 {
            tunnel: w482 -> [w485 w487]
            tunnel: [w484 w486] -> w481
            frame False {
              n225 = call "Zustandsfehlerinformation.vi"("Aktionen"=Aktionen_Zustandsfehlerinformation."Datenfehler", "String"=w485) -> ("String"=w484:string)  [unwired: 9 in]
            }
            frame True {
              n226 = flat-sequence {
                frame #0 {
                  n227 = call "FGV Erweiterte Konfig.vi"("Aktion"=FGV_PID_Aktionen."Dichtheitstest", "Dichtheitstest?"=TRUE) -> ()  [unwired: 5 in, 5 out]
                }
                frame #1 {
                  n228 = vi-ref "Erweiterte Konfig.lvlib:Dichtheitstest.vi"() -> (w491:refnum<vi>)
                  n229 = call "VI Pop Up.vi"("VI Referenz"=w491) -> ()  [unwired: 11 in]
                }
              }
              n230 = call "Zustandsfehlerinformation.vi"("Aktionen"=Aktionen_Zustandsfehlerinformation."OK", "String"=w487) -> ("String"=w486:string)  [unwired: 9 in]
            }
          }
        }
      }
    }
  }
  "String für schreiben" <- w5
  n231 = disable-structure shown="Deaktiviert" {
    frame Disabled {
      n232 = call "Gespeicherte Werte.vi"("Aktionen"=Aktionen_Gespeicherte_Werte."lesen") -> ("AKTIV?"=w492:bool[])  [unwired: 6 in, 4 out]
      n233 = Index Array(array=w492, index=3 ("Index")) -> (element=w495:bool)
      n234 = case shown="True" w495 {
        tunnel: [w496 w517] -> _
        tunnel: [_ w516] -> _
        frame True {
          n235 = for {
            tunnel: [w506] -> w496 mode=indexing
            shift-right: [w509] -> _
            shift-left: "" -> [w508]
            tunnel: _ -> [w507]
            i -> [w499]
            n236 = Index Array(array=w507, index=w506) -> (element=w504)
            n237 = for {
              N: 15 -> [_]
              shift-right: [w514] -> w503
              shift-left: w504 -> [w515]
              stop <- w512 stop-if-true
              n238 = call <vilib>:"Space Constant.vi"() -> ("String"=w511:string)
              n239 = Search and Replace String(input string=w515, search string=w511, replace string="_") -> (result string=w514:string, number of replacements=w513:i32)  [unwired: 5 in, 2 out]
              n240 = Less Or Equal To 0?(x=w513) -> (x <= 0?=w512:bool)
            }
            n241 = Increment(x=w499) -> (x+1=w501:i32)
            n242 = Number To Decimal String(number=w501) -> (decimal integer string=w498:string)  [unwired: 1 in]
            n243 = call <vilib>:"Space Constant.vi"() -> ("String"=w502:string)
            n244 = Concatenate Strings(w508, w502, w503, w502, "K" ("String"), w498) -> (w509:string)
          }
        }
        frame False {
          n245 = for {
            tunnel: w517 -> [w522] mode=indexing
            shift-right: [w529] -> w516
            shift-left: "" -> [w528]
            i -> [w524]
            n246 = Number To Decimal String(number=w522) -> (decimal integer string=w520:string)  [unwired: 1 in]
            n247 = Concatenate Strings("Gas" ("String"), w520) -> (w519:string)
            n248 = Increment(x=w524) -> (x+1=w526:i32)
            n249 = Number To Decimal String(number=w526) -> (decimal integer string=w523:string)  [unwired: 1 in]
            n250 = call <vilib>:"Space Constant.vi"() -> ("String"=w527:string)
            n251 = Concatenate Strings(w528, w527, w519, w527, "K" ("String"), w523) -> (w529:string)
          }
        }
      }
    }
    frame Enabled {
    }
  }
  n252 = disable-structure shown="Deaktiviert" {
    frame Disabled {
      n253 = call "Gespeicherte Werte.vi"("Aktionen"=Aktionen_Gespeicherte_Werte."lesen") -> ("AKTIV?"=w533:bool[])  [unwired: 6 in, 4 out]
      n254 = Index Array(array=w533, index=3 ("Index")) -> (element=w530:bool)
      n255 = case shown="True" w530 {
        tunnel: _ -> [w534 w546]
        tunnel: [w535 w545] -> _
        tunnel: _ -> [_ w544]
        tunnel: [w536 w543] -> _
        frame False {
          # "AK Standard (Gas1 Gas5)"
          n256 = for {
            tunnel: w534 -> [w541] mode=indexing
            tunnel: [w540] -> w535 mode=indexing
            tunnel: [w537] -> w536
            stop <- w537 stop-if-true
            # "kleiner als 4 = Fehler!!"
            n257 = Decimal String To Number(string=w541, offset=3 ("Offset")) -> (offset past number=w538:i32, number=w540:i32)  [unwired: 1 in]
            n258 = Less?(x=w538, y=4) -> (x < y?=w537:bool)
          }
        }
        frame True {
          # "AK Namen verwenden!!"
          n259 = for {
            tunnel: w546 -> [w549] mode=indexing
            tunnel: [w548] -> w545 mode=indexing
            tunnel: w544 -> [w550]
            tunnel: [w551] -> w543
            stop <- w551 stop-if-true
            n260 = call "String suchen AK.vi"("gesucht"=w549, "Namen"=w550) -> ("Index"=w548:i32, "Gefunden?"=w547:bool)  [unwired: 8 in]
            n261 = Not(x=w547) -> (.not. x?=w551:bool)
          }
        }
      }
    }
    frame Enabled {
    }
  }
